vi "Sequence.PopulateMCL.vi"(8 "error in (no error)":errorcluster, 10 "Sequence Data":T1[](array[typedef]), 11 "MCListbox Refnum":refnum<vi>) -> (0 "error out":errorcluster)   [LabVIEW 2019]
doc: "Populates a multi-column listbox (MCL) table with the sequence data in a tabular format."
uses:
  typedefs/step.data--Cluster.ctl
  typedefs/step.IO.data--Cluster.ctl
  typedefs/IOType--Enum.ctl
panel:
  in  "Recipe (Debug)":i32(listbox)
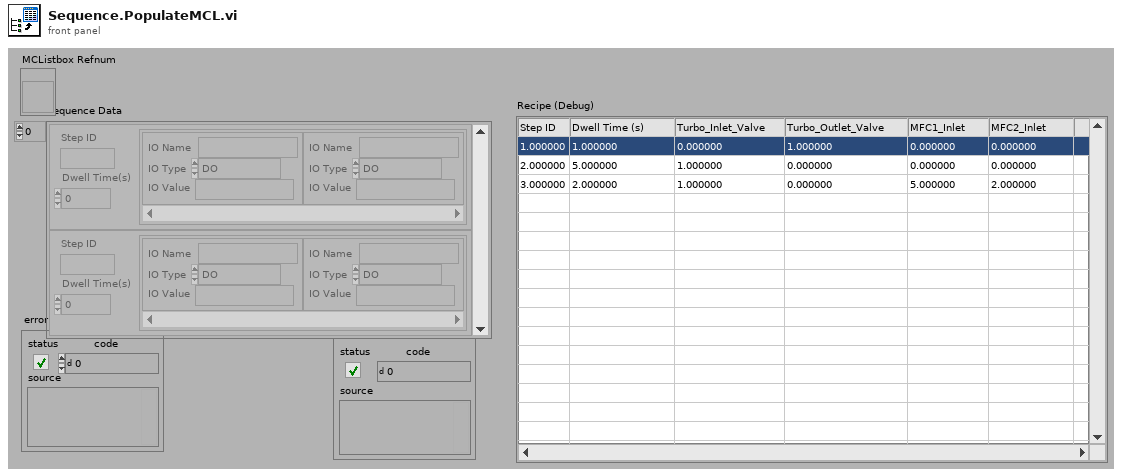
[diagram p1: front panel]
types:
  T1 = typedef "step.data--Cluster.ctl" = cluster{"Step ID":string, "Dwell Time(s)":dbl, "Recipe Step":T2[]}
  T2 = typedef "step.IO.data--Cluster.ctl" = cluster{"IO Name":string, "IO Type":T3, "IO Value":variant}
  T3 = typedef "IOType--Enum.ctl" = enum16{"<Undefined>", "DO", "DI", "AO", "AI"}
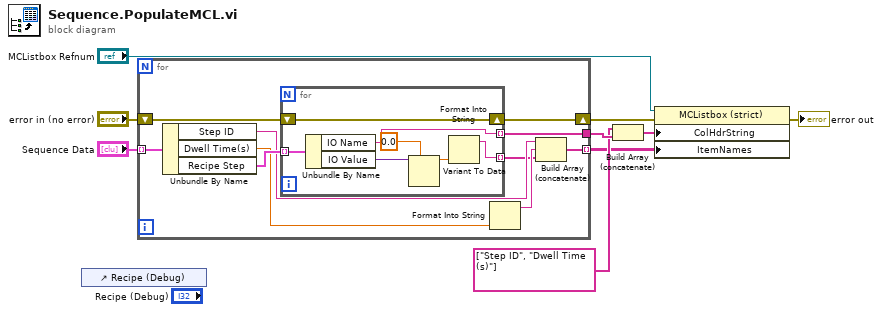
[diagram p0: block diagram]
diagram:
  n1 = control-ref of="Recipe (Debug)"() -> ()  [unwired: 1 out]
  n2 = for {
    tunnel: "Sequence Data" -> [w19] mode=indexing
    tunnel: [w17] -> w7
    shift-right: [w16] -> w4
    shift-left: "error in (no error)" -> [w15]
    tunnel: [w10] -> w2 mode=indexing
    n3 = Unbundle By Name(w19) -> ("Step ID"=w12:string, "Dwell Time(s)"=w14:dbl, "Recipe Step"=w18:T2[])
    n4 = for {
      tunnel: w18 -> [w26] mode=indexing
      tunnel: [w25] -> w17 mode=indexing
      shift-right: [w24] -> w16
      shift-left: w15 -> [w24]
      tunnel: [w20] -> w11 mode=indexing
      n5 = Unbundle By Name(w26) -> ("IO Name"=w25:string, "IO Value"=w23:variant)
      n6 = Variant To Data(type=0.0, Variant=w23) -> (data=w21:dbl)  [unwired: 1 in, 1 out]
      n7 = Format Into String(w21) -> (resulting string=w20:string)  [unwired: 3 in, 1 out]
    }
    n8 = Format Into String(w14) -> (resulting string=w13:string)  [unwired: 3 in, 1 out]
    n9 = Build Array (concatenate)(w12, w13, w11) -> (w10:string[])
  }
  n10 = Build Array (concatenate)(string[] ["Step ID", "Dwell Time (s)"], w7) -> (w5:string[])
  n11 = property class="MCListbox (strict)"(reference="MCListbox Refnum", error in=w4, "ColHdrString"=w5, "ItemNames"=w2) -> (error out=→"error out":errorcluster)  [unwired: 1 out]
